vi "latch_dram_readout.vi"(9 "Reset":bool, 10 "Output Valid":bool, 11 "Data":bool[](array[boolean])) -> (1 "Lateched Output Valid":bool, 2 "latched U64 1":u64, 3 "lateched U64 0":u64)   [LabVIEW 2014]
doc: "Latches DRAM read as two U64 and the output valid bool of the DRAM retrieve data. \nThe U64 are used as input to the DMA."
uses:
  <instrlib>/_niInstr/Basic Elements/v1/FPGA/Private/D Latch U64.vi
  <instrlib>/_niInstr/Basic Elements/v1/FPGA/niInstr Basic Elements v1 FPGA.lvlib
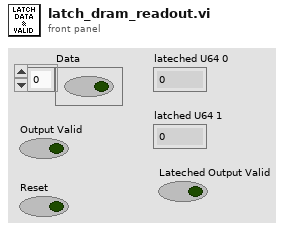
[diagram p1: front panel]
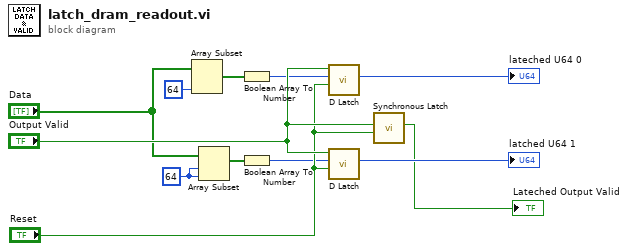
[diagram p0: block diagram]
diagram:
  w7 = 64 ("index")
  n1 = Array Subset(array="Data", length=64 ("index")) -> (w1:bool[])  [unwired: 1 in]
  n2 = Array Subset(array="Data", index=w7, length=w7) -> (w5:bool[])
  n3 = Boolean Array To Number(Boolean array=w1) -> (number=w3:u64)
  n4 = Boolean Array To Number(Boolean array=w5) -> (number=w6:u64)
  n5 = call-poly <instrlib>:"D Latch.vi"("r"="Reset", "d"=w3, "s"="Output Valid") -> ("q"=→"lateched U64 0":u64)  [unwired: 8 in]
  n6 = call-poly <instrlib>:"D Latch.vi"("r"="Reset", "d"=w6, "s"="Output Valid") -> ("q"=→"latched U64 1":u64)  [unwired: 8 in]
  n7 = call <instrlib>:"Synchronous Latch.vi"("clear"="Reset", "set"="Output Valid") -> ("out"=→"Lateched Output Valid":bool)  [unwired: 9 in]
